vi "_getDataFromFlattenedString.vi"(6 "type descriptor":variant, 8 "error in (no error)":errorcluster, 9 "offset to extract data":i32, 11 "flattened data":string) -> (0 "error out":errorcluster, 1 "offset past data":i32, 3 "data":variant)   [LabVIEW 2013, in "BSON.lvlib" / "tBSONDocument.lvclass"]
doc: "Retrieves a variant with data from a given offset in a flattened string of data."
uses:
  tBSONDocument.lvclass
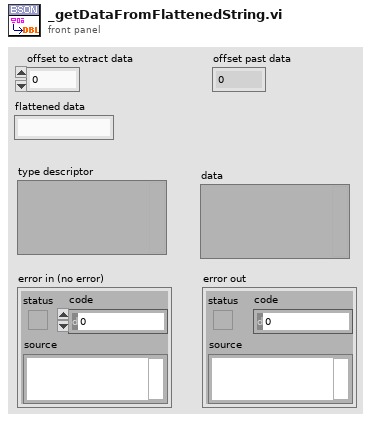
[diagram p1: front panel]
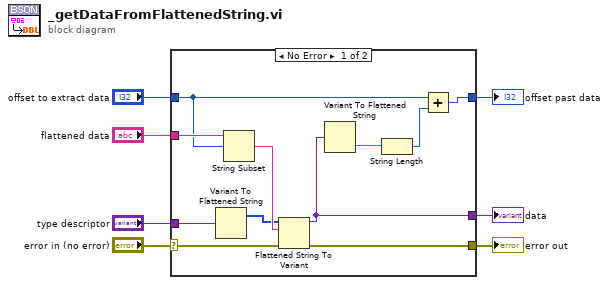
[diagram p0: block diagram]
diagram:
  n1 = case shown="No Error" "error in (no error)" {
    selector: "error in (no error)" -> [w8 w20]
    tunnel: [w18 _] -> w7
    tunnel: [w17 w20] -> w6
    tunnel: "flattened data" -> [w14 _]
    tunnel: "type descriptor" -> [w13 _]
    tunnel: "offset to extract data" -> [w11 w19]
    tunnel: [w9 w19] -> w2
    frame No Error {
      n2 = Variant To Flattened String(Variant=w13) -> (1:w15:i16[])  [unwired: 1 out]
      n3 = String Subset(string=w14, offset (0)=w11) -> (substring=w16:string)  [unwired: 1 in]
      n4 = Flattened String To Variant(4:w8, 6:w16, 7:w15) -> (0:w17:errorcluster, 3:w18:variant)
      n5 = Variant To Flattened String(Variant=w18) -> (data string=w12:string)  [unwired: 1 out]
      n6 = String Length(string=w12) -> (length=w10:i32)
      n7 = Add(x=w11, y=w10) -> (x+y=w9:i32)
    }
    frame Error {
    }
  }
  "data" <- w7
  "error out" <- w6
  "offset past data" <- w2
